vi "Parse Digital Line.vi"(4 "Resource String":string) -> (7 "Digital Channel":T1)   [LabVIEW 2020, in "VolatusDAQ.lvlib" / "DAQmxDI.lvclass"]
uses:
  DAQmxDI.lvclass
  Digital Line.ctl
  DAQmxDI.lvclass/DAQmxDI.ctl
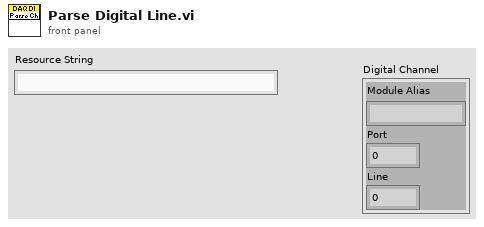
[diagram p1: front panel]
types:
  T1 = typedef "VolatusDAQ.lvlib/DAQmxDI.lvclass/Digital Line.ctl" = cluster{"Module Alias":string, "Port":i32, "Line":i32}
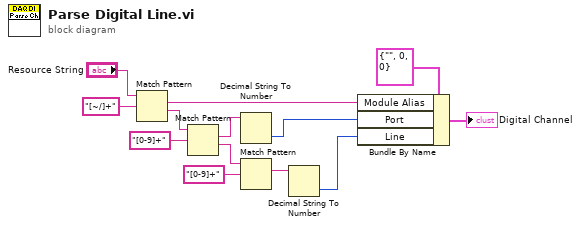
[diagram p0: block diagram]
diagram:
  n1 = Match Pattern(string="Resource String", regular expression="[~/]+") -> (match substring=w10:string, after substring=w7:string)  [unwired: 1 in, 2 out]
  n2 = Match Pattern(string=w7, regular expression="[0-9]+") -> (match substring=w6:string, after substring=w3:string)  [unwired: 1 in, 2 out]
  n3 = Decimal String To Number(string=w6) -> (number=w5:i32)  [unwired: 2 in, 1 out]
  n4 = Match Pattern(string=w3, regular expression="[0-9]+") -> (match substring=w2:string)  [unwired: 1 in, 3 out]
  n5 = Decimal String To Number(string=w2) -> (number=w1:i32)  [unwired: 2 in, 1 out]
  n6 = Bundle By Name(cluster=T1 {"Module Alias"="", "Port"=0, "Line"=0} ("Digital Channel"), "Module Alias"=w10, "Port"=w5, "Line"=w1) -> (→"Digital Channel":T1)
